vi "availablePlaces.vi"(8 "pos":i32[][](array[numeric]), 9 "exist":i32[][](array[numeric]), 10 "available":i32[][](array[numeric]), 11 "redTurn":i32) -> (0 "posNew":i32[][](array[numeric]), 1 "existNew":i32[][](array[numeric]), 2 "availableNew":i32[][](array[numeric]), 3 "count":i32)   [LabVIEW 2022 SP3, in "subvis.lvlib"]
uses:
  subvis.lvlib
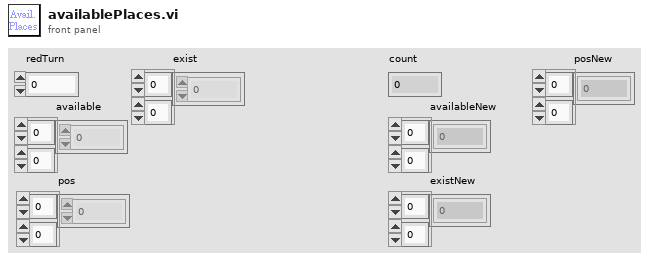
[diagram p1: front panel]
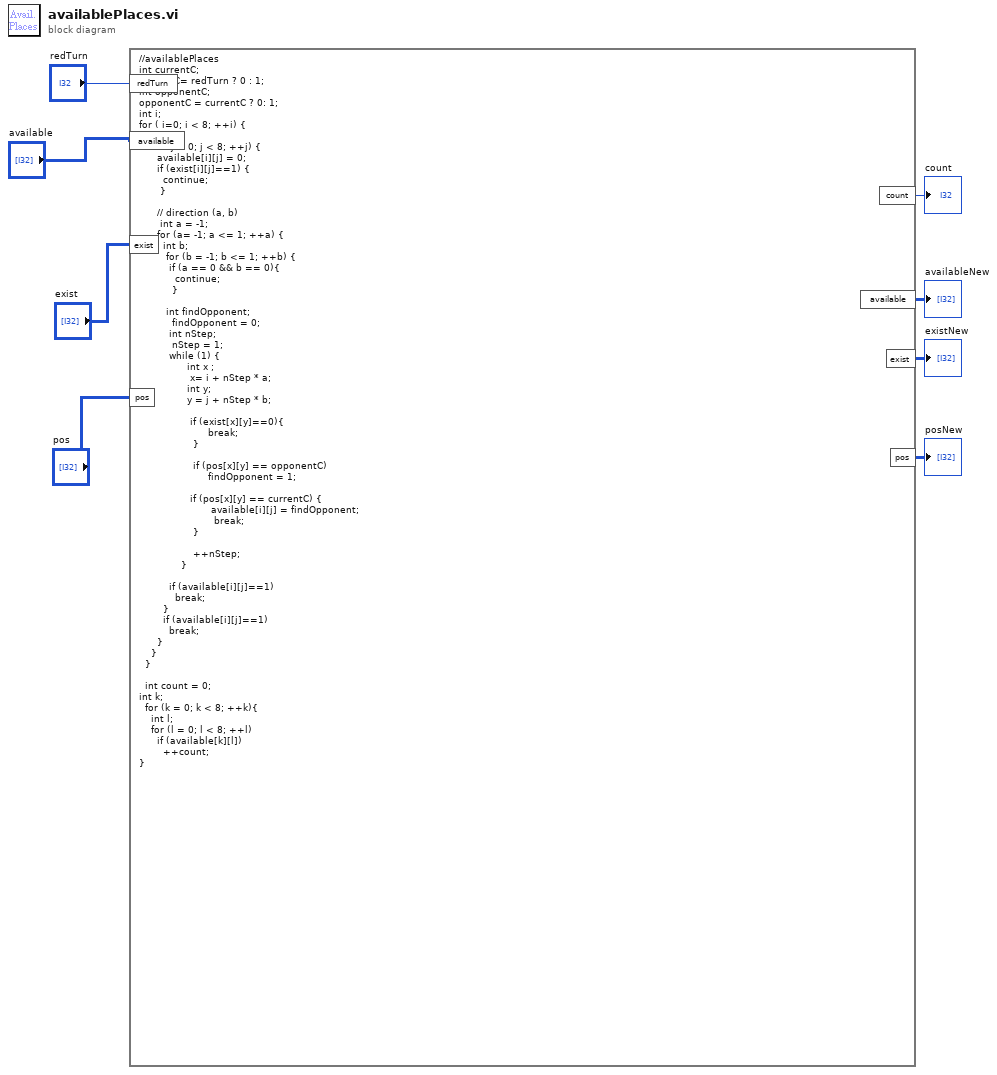
[diagram p0: block diagram]
diagram:
  n1 = formula code="//availablePlaces\nint currentC; \ncurrentC= redTurn ? 0 : 1;\nint opponentC;\nopponentC = currentC ? 0: 1;\nint i;\nfor ( i=0; i < 8; ++i) {\nint j;\n    for (j = 0; j < 8; ++j) {\n      available[i][j] = 0;\n      if (exist[i][j]==1) {\n        continue;\n       }\n\n      // direction (a, b)\n       int a = -1;       \n      for (a= -1; a <= 1; ++a) {\n        int b;\n         for (b = -1; b <= 1; ++b) {\n          if (a == 0 && b == 0){\n            continue;\n           }\n\n         int findOpponent;\n           findOpponent = 0;\n          int nStep;\n           nStep = 1;\n          while (1) {\n                int x ;\n                 x= i + nStep * a;\n                int y;\n                y = j + nStep * b;\n        \n                 if (exist[x][y]==0){\n                       break;\n                  }\n\n                  if (pos[x][y] == opponentC)\n                       findOpponent = 1;\n\n                 if (pos[x][y] == currentC) {\n                        available[i][j] = findOpponent;\n                         break;\n                  }\n\n                  ++nStep;\n              }\n\n          if (available[i][j]==1)\n            break;\n        }\n        if (available[i][j]==1)\n          break;\n      }\n    }\n  }\n\n  int count = 0;\nint k;\n  for (k = 0; k < 8; ++k){\n    int l;\n    for (l = 0; l < 8; ++l)\n      if (available[k][l])\n        ++count;\n}"("available"="available", "exist"="exist", "pos"="pos", "redTurn"="redTurn") -> ("count"=→"count":i32, "available"=→"availableNew":i32[][], "exist"=→"existNew":i32[][], "pos"=→"posNew":i32[][])
